vi "Sample Orders from Order Spe.vi"(2 "Order info":cluster{"min":dbl, "resolution":dbl} {"resolution" format="%.2f"; "min" format="%.2f"}, 3 "order spectrum":u8[][](array[numeric])) -> (0 "Order array":dbl[](array[numeric]) format="%.2f")   [LabVIEW 2017]
uses:
  <vilib>/Analysis/1siggen.llb/Ramp Pattern by Samples.vi
  <vilib>/Analysis/NI_AALBase.lvlib
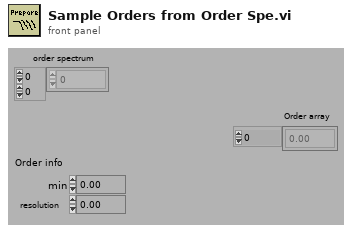
[diagram p1: front panel]
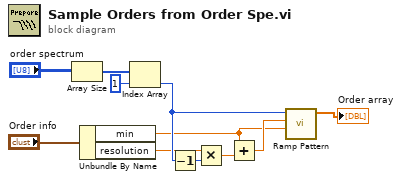
[diagram p0: block diagram]
diagram:
  n1 = Array Size(array="order spectrum") -> (size(s)=w11:i32[])
  n2 = Unbundle By Name("Order info") -> ("min"=w1:dbl, "resolution"=w5:dbl)
  n3 = Index Array(array=w11, index=1 ("Index")) -> (element=w6:i32)
  n4 = Decrement(x=w6) -> (x-1=w4:i32)
  n5 = Multiply(x=w5, y=w4) -> (x*y=w3:dbl)
  n6 = Add(x=w1, y=w3) -> (x+y=w2:dbl)
  n7 = call-poly <vilib>:"Ramp Pattern.vi"("start"=w1, "end"=w2, "samples"=w6) -> ("Ramp Pattern"=→"Order array":dbl[])  [unwired: 7 in, 1 out]
